vi "New Panel UE Handle.vi"(8 "error in (no error)":errorcluster, 10 "NewPanel":T1, 11 "TipPanel in":refnum<class "TipPanel.lvclass">) -> (0 "error out":errorcluster, 1 "Promise.Size":refnum<class "Promise.lvclass">, 2 "DATA ONLY":refnum<class "TipPanel.lvclass">)   [LabVIEW 2021, in "TipStripOOPanel.lvlib" / "TipPanel.lvclass"]
uses:
  TipPanel.lvclass
  ToPanelUE.ctl
  <vilib>/Futures/Futures/Promise/Promise.lvclass
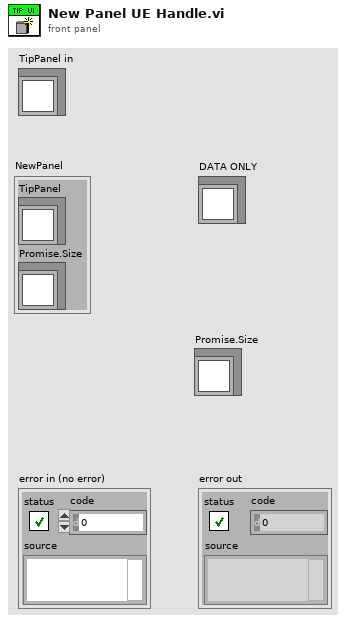
[diagram p1: front panel]
types:
  T1 = typedef "TipStripOOPanel.lvlib/TipPanel.lvclass/ToPanelUE.ctl" = cluster{"TipPanel":refnum<class>, "Promise.Size":refnum<class "Promise.lvclass">}
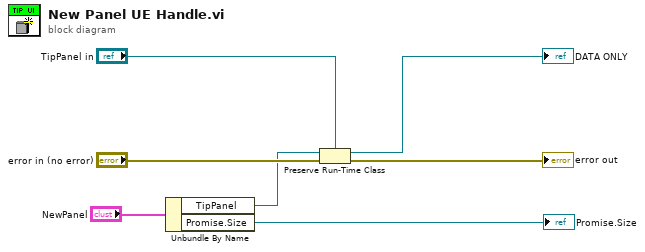
[diagram p0: block diagram]
diagram:
  n1 = Unbundle By Name("NewPanel") -> ("TipPanel"=w2:refnum<class>, "Promise.Size"=→"Promise.Size":refnum<class "Promise.lvclass">)
  n2 = Preserve Run-Time Class(object in=w2, error in="error in (no error)", 2:"TipPanel in") -> (object out=→"DATA ONLY":refnum<class "TipPanel.lvclass">, error out=→"error out":errorcluster)
